vi "Modbus Value to data stream.vi"(4 "register values":u16[](array[numeric])) -> (1 "String":string)   [LabVIEW 2019, in "Modbus.lvclass"]
uses:
  Modbus.lvclass
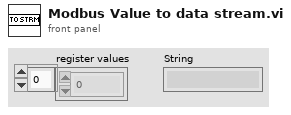
[diagram p1: front panel]
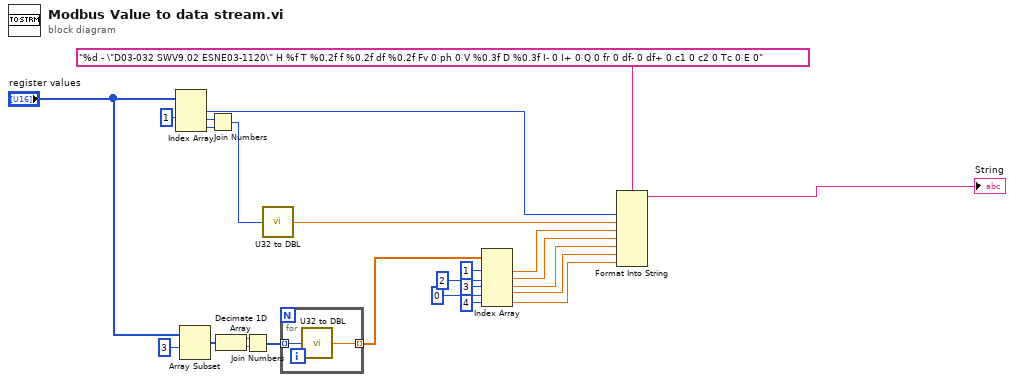
[diagram p0: block diagram]
diagram:
  n1 = Index Array(array="register values", index #2=1 ("index")) -> (element #1=w15:u16, element #2=w3:u16, element #3=w2:u16)  [unwired: 2 in]
  n2 = Array Subset(array="register values", index=3) -> (w7:u16[])  [unwired: 1 in]
  n3 = Join Numbers(hi=w3, lo=w2) -> ((hi.lo)=w4:u32)
  n4 = Decimate 1D Array(w7) -> (w8:u16[], w9:u16[])
  n5 = Join Numbers(hi=w8, lo=w9) -> ((hi.lo)=w10:u32[])
  n6 = call "U32 to DBL.vi"("U32"=w4) -> ("DBL"=w13:dbl)  [unwired: 6 in]
  n7 = for {
    tunnel: w10 -> [w27] mode=indexing
    tunnel: [w26] -> w12 mode=indexing
    n8 = call "U32 to DBL.vi"("U32"=w27) -> ("DBL"=w26:dbl)  [unwired: 6 in]
  }
  n9 = Index Array(array=w12, index #1=1 ("index"), index #2=2 ("index"), index #3=3 ("index"), index #4=0 ("index"), index #5=4 ("index")) -> (element #1=w16:dbl, element #2=w17:dbl, element #3=w19:dbl, element #4=w21:dbl, element #5=w24:dbl)
  n10 = Format Into String(format string="%d - \"D03-032 SWV9.02 ESNE03-1120\" H %f T %0.2f f %0.2f df %0.2f Fv 0 ph 0 V %0.3f D %0.3f I- 0 I+ 0 Q 0 fr 0 df- 0 df+ 0 c1 0 c2 0 Tc 0 E 0", w15, w13, w16, w17, w19, w21, w24) -> (resulting string=→"String":string)  [unwired: 2 in, 1 out]
